vi "ScanTrans.vi"(0 "Type of scan":u16(ring)=3 items=["Therapy With Scan", "M scan", "M Scan With Therapy Burst", "1-D B Scan", "1-D B Scan With Therapy Burst", "2-D B Scan", "2-D B Scan With Therapy Burst", "Rotational Scan", "1-D B-Scan PRF", "2-D B-Scan PRF", "Real-Time Scan", "Contrast Agents", "1-D w/ Real-Time Set Up", "Amplifier blah blah"], 1 "File Name":string, 2 "Digitizer Settings":T5={"Digitizer delay (us) "=0.0, "rf points per line"=2048, "lines per plane"=128, "Samp Rate (Hz)"=100000000.0, "Additional dig delay (us)"=0.0, "Voltage Scale"=0.4, "Pre-Looks"=0, "Offset delay (us)"=0.0, "bits A/D"=8, "Avg Num"=1, "DigTimeOut"=5.0, "Rel Dig Delay"=0.0, "Dig Ch"=0, "LeCroyCluster"={"LeCroy Channels"=[TRUE, FALSE, FALSE, FALSE], "LC read pt offset"=0.0, "Sweep Avg"=FALSE}, "Main Digitizer"=enum."NI Digitizer", "Dig Config"=enum."Single channel", "Digitizer ID Cluster"={"Acqiris/Alazar/SP ID"=[], "NI Instr Handles"=[], "LeCroy VISA"="", "GaGe Handle"={"Handle"=0, "Sample size"=0, "Resolution"=0, "Offset"=0, "Channels"=0, "Boards"=0}, "ATS Ref"="ATS9350", "Acqiris Address"=["PCI::INSTR0"], "ADQRef"=refnum, "adq_cu_ptr"=refnum}, "Trigger Settings"={"Trig Source"=1, "Trig Coupling"=0, "Trig Slope"=0, "Level (mV)"=1500.0}, "Bulk Acq"=FALSE, "Bulk Start Indexes"=[], "Data Ref RF"=refnum, "NI ID/Channel"=[], "Total Dig CH"=5, "Xtra Ann Trig delay (us)"=10.0, "Fix Z Delay?"=FALSE, "One Way Transmission?"=FALSE, "Data Ref Log"=refnum} {"Trigger Settings"."Trig Slope" items=["Positive", "Negative"]; "Trigger Settings"."Level (mV)" format="%.2f"; "Trigger Settings"."Trig Coupling" items=["DC 1 MOhm", "AC 1 MOhm", "DC 50 Ohm", "AC 50 Ohm"]; "Trigger Settings"."Trig Source" items=["Chan 1", "External"]; "Rel Dig Delay" format="%.2f"; "DigTimeOut" format="%.2f"; "Avg Num" min=1; "Offset delay (us)" format="%.2f"; "Additional dig delay (us)" format="%.2f"; "Digitizer delay (us)" format="%.2f"}, 5 "Scan Length (mm)":dbl=10.0 format="%.2f", 7 "Therapy":bool, 12 "Motion Settings":T1={"No Motion?"=FALSE, "Motion System"=enum."No Motion Card", "Motion Bd ID"=1, "Motion Profile"="SMAC1", "# Axis"=1, "Reverse Z axis?"=TRUE, "SMAC Axis"=0, "scan pair"=enum."y-(x) scan", "RT fps"=6.0, "Steps per mm"=[1000, 1000, 1000, 1000], "Motor Parameters"={"velocity ct/s"=[10000.0, 10000.0, 10000.0, 50000.0], "accel ct/s^2"=[50000.0, 50000.0, 50000.0, 200000.0]}, "One Way Scan"=FALSE, "Reverse One Way Scan"=FALSE, "Global Position (mm)"=[], "Plane"=0, "Distance between\nscan lines (um)"=0.0, "Distance between\nscan planes (um)"=0.0, "number of scan planes"=1, "Total steps in line"=0, "Xtra plane\ndistance  (um)"=100, "Xtra planes "=1, "Add Axis"=FALSE, "overshoot cts"=200, "BKPT Shift"=0, "Scan Start Time (ms)"=0, "ESP VISA"="GPIB::1::INSTR", "3rd Axis"=1, "GL Ref Out"=refnum, "Galil Address"=""} {"3rd Axis" items=["x", "y", "z", "w"]; "Xtra planes" min=1; "Xtra plane\ndistance  (um)" min=0; "Distance between\nscan planes (um)" format="%.2f"; "Distance between\nscan lines (um)" format="%.2f"; "SMAC Axis" items=["None"=0, "Axis 1"=1, "Axis 2"=2, "Axis 3"=3, "Axis 4"=4, "Axis 5"=5, "Axis 6"=6, "Axis 7"=7, "Axis 8"=8, "Vector Space 1"=17, "Vector Space 2"=18, "Vector Space 3"=19, "Vector Space 4"=20]; "Motion Bd ID" min=1 max=32 step=1}, 14 "Pressure Cal Parameters":T9={"Center Freq (MHz)"=0.0, "PRF (kHz)"=0.0, "Pulse window (us)"=0.0, "Hydrophone"=enum."PAL #1048", "booster amp?"=TRUE} {"Pulse window (us)" format="%.2f"; "PRF (kHz)" format="%.2f"; "Center Freq (MHz)" format="%.2f"}) -> (4 "Scan data":T11 {"Pulse Parameters"."pos peak pressure (MPa)" format="%.2f"; "axis 2 ticks" format="%.2f"; "axis 1 ticks" format="%.2f"; "step size" format="%.2f"; "axis2o" format="%.2f"; "axis1o" format="%.2f"; "scan data" format="%.2f"})   [LabVIEW 2022 SP3]
uses:
  HydrophoneSettings.ctl
  Hydros.ctl
  ScanningControl/Digitizers/-DigitizerRoutines/DigitizerSettings.ctl
  ScanningControl/Digitizers/-DigitizerRoutines/Digitizer.ctl
  ScanningControl/Digitizers/-DigitizerRoutines/DigConfig.ctl
  ScanningControl/Digitizers/-DigitizerRoutines/DigitizerID.ctl
  C:/Windows/System32/ADQAPI_dotNet_helper.dll
  ScanningControl/Motion Controllers/NI_controller/-NI_MotionRoutines/MotionParameters.ctl
  ScanningControl/Motion Controllers/NI_controller/-NI_MotionRoutines/MotionSys.ctl
  ScanningControl/Motion Controllers/-MotionRoutines/ScanAxis.ctl
  ScanningControl/Motion Controllers/-MotionRoutines/3rdAxis.ctl
  ScanningControl/Motion Controllers/-MotionRoutines/MotionGlobals.vi
panel:
  out "Waveform Graph":dbl[](graph)
  # "1-D and 2-D B scan settings"
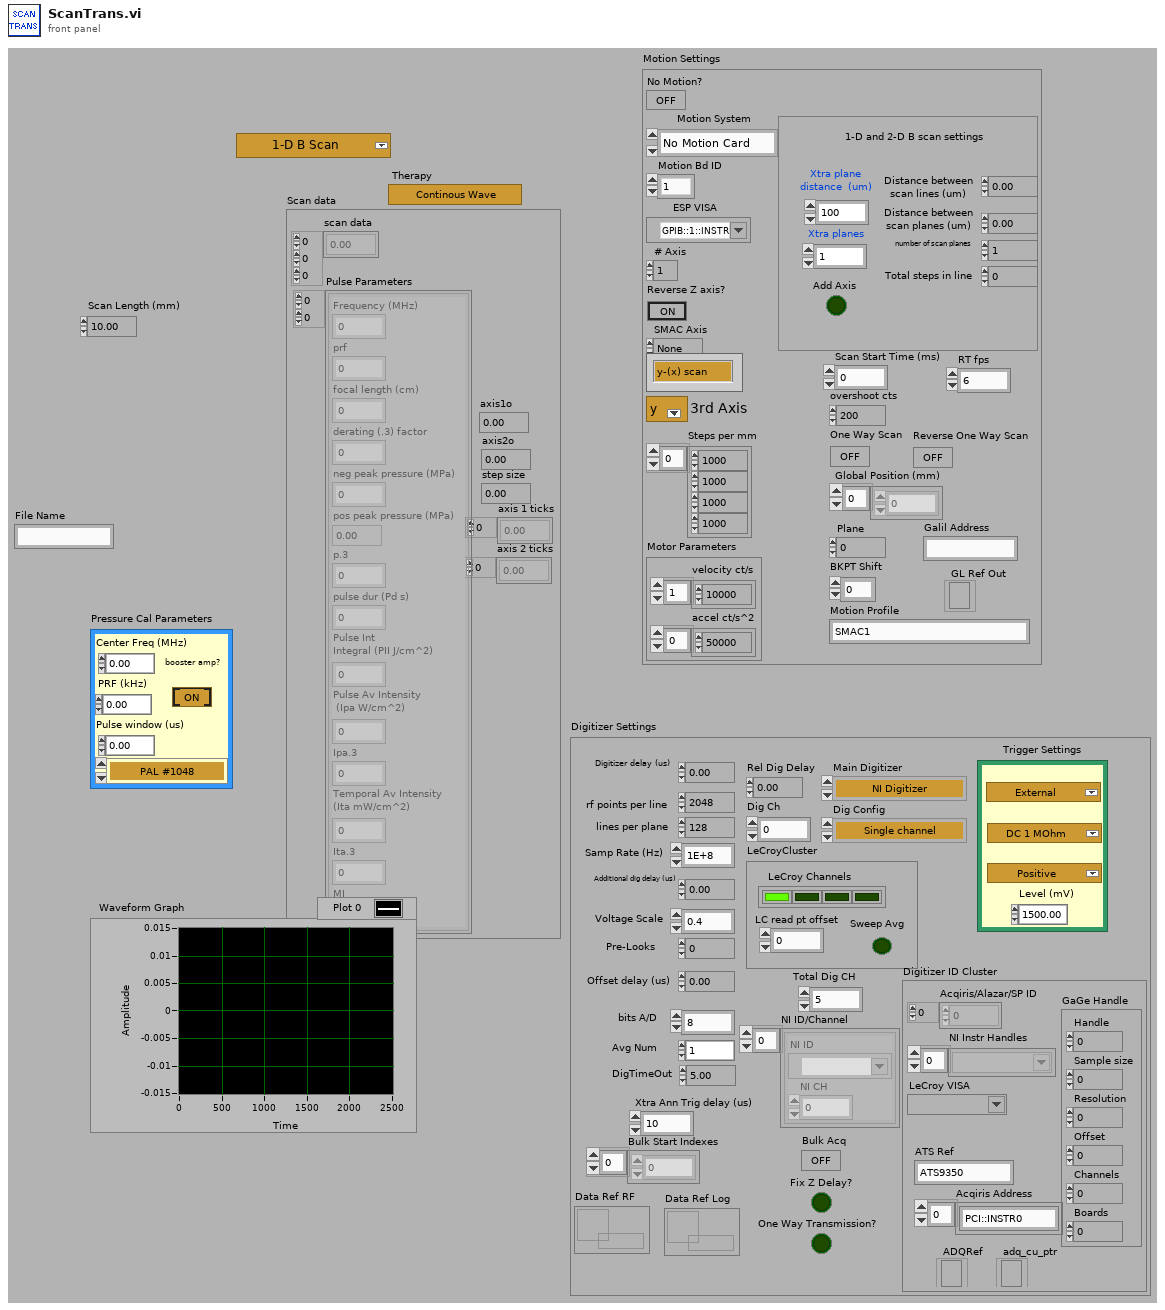
[diagram p1: front panel]
types:
  T1 = typedef "MotionParameters.ctl" = cluster{"No Motion?":bool, "Motion System":T2, "Motion Bd ID":u8, "Motion Profile":string, "# Axis":i8, "Reverse Z axis?":bool, "SMAC Axis":u16, "scan pair":T3, "RT fps":sgl, "Steps per mm":i32[], "Motor Parameters":cluster{"velocity ct/s":dbl[], "accel ct/s^2":dbl[]}, "One Way Scan":bool, "Reverse One Way Scan":bool, "Global Position (mm)":dbl[], "Plane":i32, "Distance between\nscan lines (um)":sgl, "Distance between\nscan planes (um)":sgl, "number of scan planes":i32, "Total steps in line":i32, "Xtra plane\ndistance  (um)":i32, "Xtra planes ":i32, "Add Axis":bool, "overshoot cts":i32, "BKPT Shift":i32, "Scan Start Time (ms)":u32, "ESP VISA":refnum<visa-resource-name>, "3rd Axis":T4, "GL Ref Out":refnum<k7>, "Galil Address":string}
  T2 = typedef "MotionSys.ctl" = enum16{"MM3000", "NI 735x", "Newport ESP", "No Motion Card", "Galil"}
  T3 = typedef "ScanAxis.ctl" = enum16{"y-(x) scan", "x-(y) scan", "z-(x) scan", "z-(y) scan", "y-(z) scan", "x-(z) scan", "w-(x) scan", "w-(y) scan", "w-(z) scan", "x-(w) scan", "y-(w) scan", "z-(w) scan"}
  T4 = typedef "3rdAxis.ctl" = u16
  T5 = typedef "DigitizerSettings.ctl" = cluster{"Digitizer delay (us) ":dbl, "rf points per line":i32, "lines per plane":i32, "Samp Rate (Hz)":dbl, "Additional dig delay (us)":dbl, "Voltage Scale":dbl, "Pre-Looks":i32, "Offset delay (us)":dbl, "bits A/D":i8, "Avg Num":i32, "DigTimeOut":sgl, "Rel Dig Delay":sgl, "Dig Ch":i32, "LeCroyCluster":cluster{"LeCroy Channels":bool[], "LC read pt offset":dbl, "Sweep Avg":bool}, "Main Digitizer":T6, "Dig Config":T7, "Digitizer ID Cluster":T8, "Trigger Settings":cluster{"Trig Source":u16, "Trig Coupling":u16, "Trig Slope":u16, "Level (mV)":dbl}, "Bulk Acq":bool, "Bulk Start Indexes":i32[], "Data Ref RF":refnum<data-value>, "NI ID/Channel":cluster{"NI ID":refnum<k15>, "NI CH":i32}[], "Total Dig CH":i32, "Xtra Ann Trig delay (us)":dbl, "Fix Z Delay?":bool, "One Way Transmission?":bool, "Data Ref Log":refnum<data-value>}
  T6 = typedef "Digitizer.ctl" = enum16{"Acqiris Digitizer", "NI Digitizer", "LeCroy", "GaGe", "AlazarTech", "No Digitizer", "Teledyne"}
  T7 = typedef "DigConfig.ctl" = enum16{"Single channel", "2 Chans w/ 2 Acqiris", "2 Chans w/ 1 Acqiris", "5-CH Pulser New", "5-CH pulser w/ ann array", "5-pass style ann array", "Empty"}
  T8 = typedef "DigitizerID.ctl" = cluster{"Acqiris/Alazar/SP ID":u32[], "NI Instr Handles":refnum<k15>[], "LeCroy VISA":refnum<visa-resource-name>, "GaGe Handle":cluster{"Handle":u32, "Sample size":u32, "Resolution":i32, "Offset":i32, "Channels":u32, "Boards":u32}, "ATS Ref":string, "Acqiris Address":string[], "ADQRef":refnum<k24>, "adq_cu_ptr":refnum<k24>}
  T9 = typedef "HydrophoneSettings.ctl" = cluster{"Center Freq (MHz)":dbl, "PRF (kHz)":dbl, "Pulse window (us)":dbl, "Hydrophone":T10, "booster amp?":bool}
  T10 = typedef "Hydros.ctl" = enum16{"PAL #1048", "PAL #525", "PAL #430a", "PAL #192", "DEAD PAL # 1403", "LOST UHI Onda", "DEAD PAL #1818", "PAL #1974", "DEAD #2266 w/booster", "PAL #2524 w/booster", "PAL FP21-20T", "PAL FP160-13  ", "PAL FP141-20", "PAL FP158-08T"}
  T11 = cluster{"scan data":dbl[][][], "Pulse Parameters":cluster{"Frequency (MHz)":dbl, "prf":dbl, "focal length (cm)":dbl, "derating (.3) factor":dbl, "neg peak pressure (MPa)":dbl, "pos peak pressure (MPa)":dbl, "p.3":dbl, "pulse dur (Pd s)":dbl, "Pulse Int \nIntegral (PII J/cm^2)":dbl, "Pulse Av Intensity\n (Ipa W/cm^2)":dbl, "Ipa.3":dbl, "Temporal Av Intensity \n(Ita mW/cm^2)":dbl, "Ita.3":dbl, "MI":dbl}[][], "axis1o":dbl, "axis2o":dbl, "step size":dbl, "axis 1 ticks":dbl[], "axis 2 ticks":dbl[]}
  T12 = enum16{"Absolute Position", "Relative Position", "Velocity", "Relative to Cap Pos", "Modulus Position", "Absolute Contouring", "Relative Contouring"}
  T13 = cluster{"Frequency (MHz)":dbl, "prf":dbl, "focal length (cm)":dbl, "derating (.3) factor":dbl, "neg peak pressure (MPa)":dbl, "pos peak pressure (MPa)":dbl, "p.3":dbl, "pulse dur (Pd s)":dbl, "Pulse Int \nIntegral (PII J/cm^2)":dbl, "Pulse Av Intensity\n (Ipa W/cm^2)":dbl, "Ipa.3":dbl, "Temporal Av Intensity \n(Ita mW/cm^2)":dbl, "Ita.3":dbl, "MI":dbl}[][]
  T14 = cluster{"Axis 1 Start":dbl, "Axis 2 Start":dbl, "Step Size":dbl, "Axis 1 Ticks":dbl[], "Axis 2 Ticks":dbl[]}
  T15 = cluster{dbl[][][], "Data":cluster{"Frequency (MHz)":dbl, "prf":dbl, "focal length (cm)":dbl, "derating (.3) factor":dbl, "neg peak pressure (MPa)":dbl, "pos peak pressure (MPa)":dbl, "p.3":dbl, "pulse dur (Pd s)":dbl, "Pulse Int \nIntegral (PII J/cm^2)":dbl, "Pulse Av Intensity\n (Ipa W/cm^2)":dbl, "Ipa.3":dbl, "Temporal Av Intensity \n(Ita mW/cm^2)":dbl, "Ita.3":dbl, "MI":dbl}[][], "Axis 1 Start":dbl, "Axis 2 Start":dbl, "Step Size":dbl, "Axis 1 Ticks":dbl[], "Axis 2 Ticks":dbl[]}
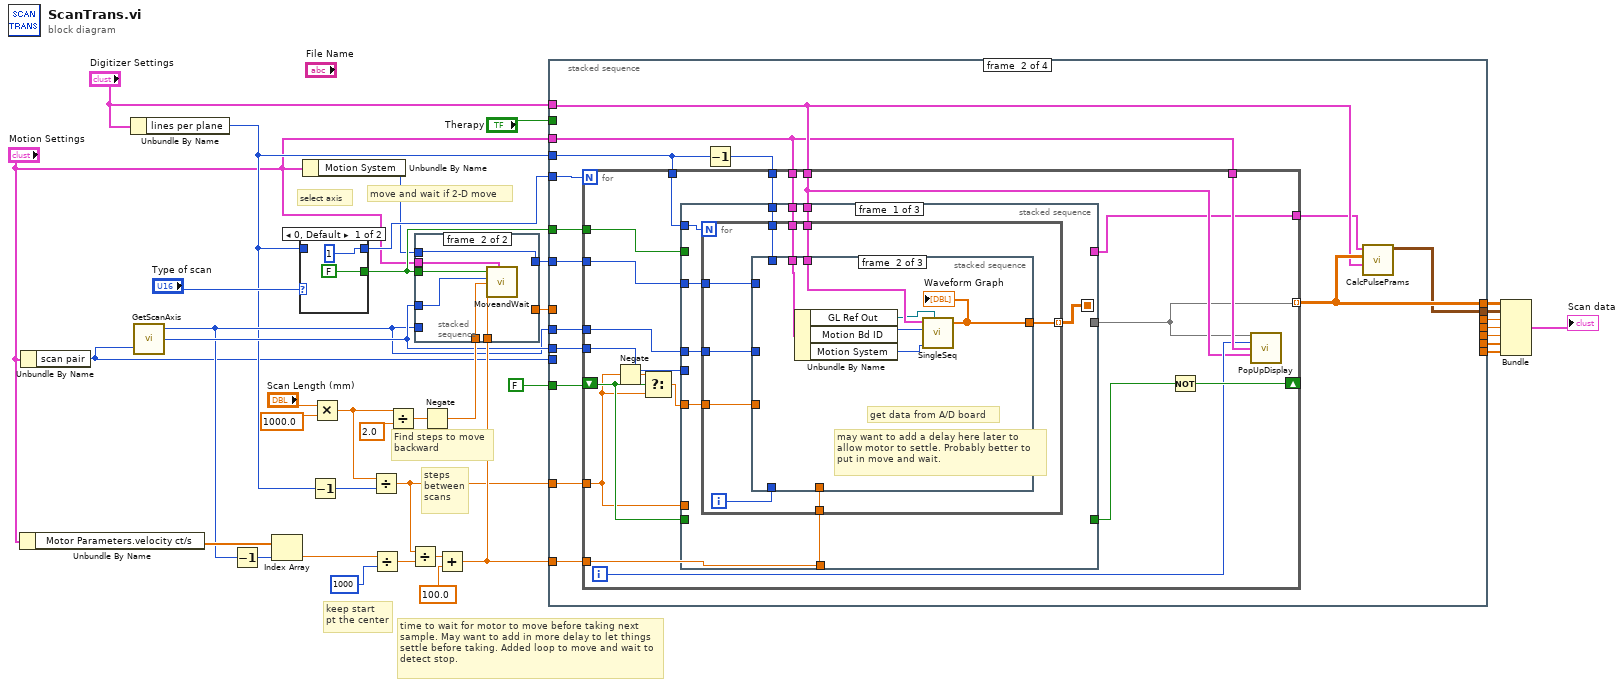
[diagram p0: block diagram]
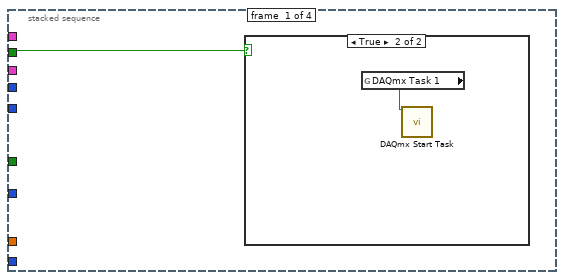
[diagram p2: hidden frame]
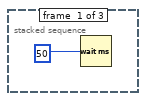
[diagram p4: hidden frame]
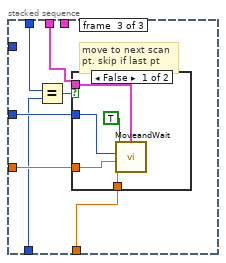
[diagram p5: hidden frame]
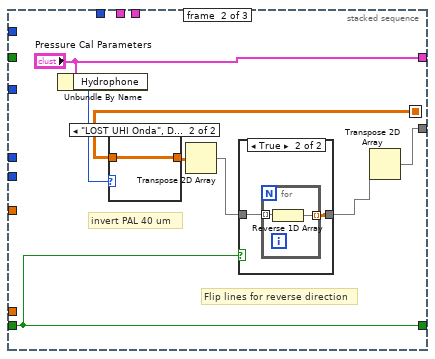
[diagram p7: hidden frame]
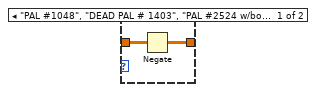
[diagram p9: hidden frame]
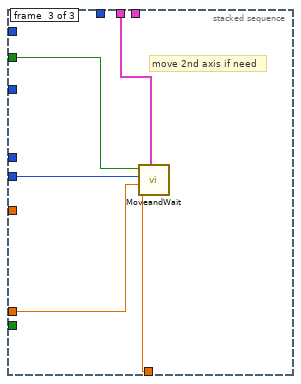
[diagram p10: hidden frame]
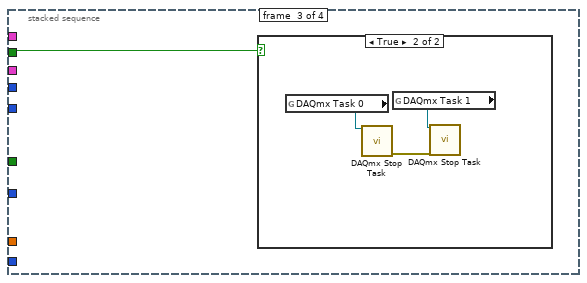
[diagram p11: hidden frame]
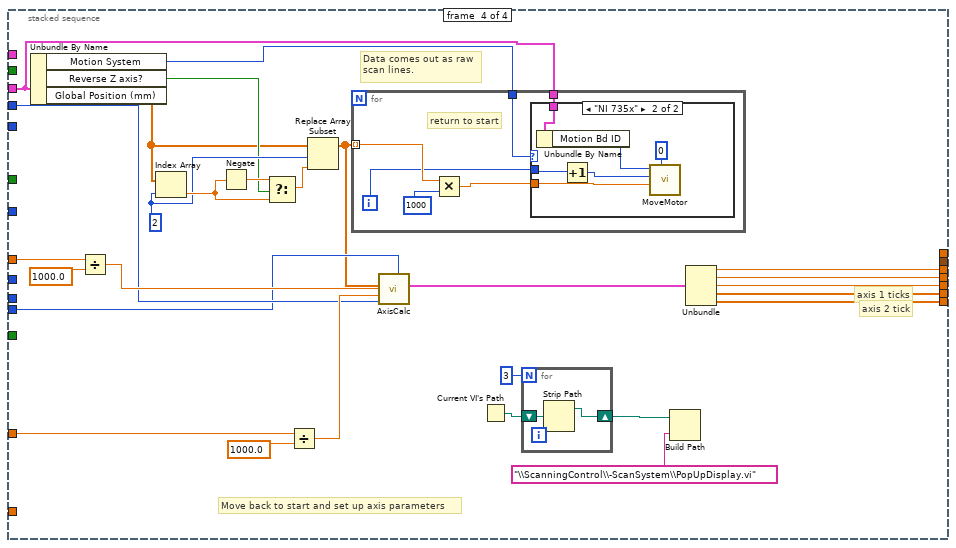
[diagram p13: hidden frame]
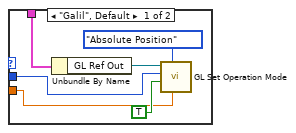
[diagram p14: hidden frame]
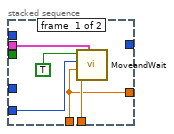
[diagram p15: hidden frame]
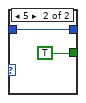
[diagram p16: hidden frame]
diagram:
  # "steps\nbetween\nscans"
  # "Find steps to move\nbackward"
  # "select axis"
  # "move and wait if 2-D move"
  # "time to wait for motor to move before taking next sample. May want to add in more delay to let things settle before taking. Added loop to move and wait to detect stop."
  # "keep start\npt the center"
  n1 = Unbundle By Name("Motion Settings") -> ("Motor Parameters.velocity ct/s"=w9:dbl[])
  n2 = Unbundle By Name("Motion Settings") -> ("scan pair"=w4:T3)
  n3 = Unbundle By Name("Digitizer Settings") -> ("lines per plane"=w5:i32)
  n4 = call "GetScanAxis.vi"("scan pair"=w4) -> ("Axis 1"=w7:i32, "Axis 2"=w11:i32)  [unwired: 1 in, 1 out]
  n5 = Decrement(x=w7) -> (x-1=w6:i32)
  n6 = Index Array(array=w9, index=w6) -> (element=w8:dbl)
  n7 = case shown="0, Default" "Type of scan" {
    tunnel: [1 w41] -> w37
    tunnel: w5 -> [_ w41]
    tunnel: [FALSE TRUE] -> w25
    frame 0, Default {
    }
    frame 5 {
      # "y"
    }
  }
  n8 = Unbundle By Name("Motion Settings") -> ("Motion System"=w3:T2)
  n9 = Decrement(x=w5) -> (x-1=w29:i32)
  n10 = Multiply(x="Scan Length (mm)", y=1000.0) -> (x*y=w30:dbl)
  n11 = Divide(x=w30, y=w29) -> (x/y=w22:dbl)
  n12 = Divide(x=w8, y=1000) -> (x/y=w27:dbl)
  n13 = Divide(x=w30, y=2.0) -> (x/y=w32:dbl)
  n14 = Divide(x=w22, y=w27) -> (x/y=w35:dbl)
  n15 = Negate(x=w32) -> (-x=w23:dbl)
  n16 = Add(x=w35, y=100.0) -> (x+y=w26:dbl)
  n17 = stacked-sequence {
    tunnel: w25 -> [_ w53]
    tunnel: w11 -> [_ w52]
    tunnel: w23 -> [w45 w51]
    tunnel: w26 -> [w46 w50]
    tunnel: w7 -> [w44 _]
    tunnel: [w45 _] -> w20
    tunnel: w3 -> [_ w49]
    tunnel: [_ w49] -> w19
    tunnel: "Motion Settings" -> [w43 w48]
    frame #0 {
      n18 = call "MoveandWait.vi"("Motion Settings"=w43, "time to wait (ms)"=w46, "steps to move"=w45, "Axis"=w44, "Move and Wait?"=TRUE) -> ()  [unwired: 1 in, 2 out]
    }
    frame #1 {
      n19 = call "MoveandWait.vi"("Motion Settings"=w48, "time to wait (ms)"=w50, "steps to move"=w51, "Axis"=w52, "Move and Wait?"=w53) -> ()  [unwired: 1 in, 2 out]
    }
  }
  n20 = stacked-sequence {
    tunnel: w37 -> [_ w70 _ _]
    tunnel: FALSE -> [_ w69 _ _]
    tunnel: w26 -> [_ w67 _ _]
    tunnel: w7 -> [_ w66 _ _]
    tunnel: w25 -> [_ w65 _ _]
    tunnel: w11 -> [_ w64 _ _]
    tunnel: w22 -> [_ w63 _ w176]
    tunnel: [_ w60 _ _] -> w24
    tunnel: w5 -> [_ w62 _ w165]
    tunnel: [_ w59 _ _] -> w21
    tunnel: w20 -> [_ _ _ w174]
    tunnel: w19 -> [_ w61 _ _]
    tunnel: [_ _ _ w172] -> w18
    tunnel: [_ _ _ w171] -> w17
    tunnel: [_ _ _ w170] -> w16
    tunnel: [_ _ _ w169] -> w15
    tunnel: [_ _ _ w168] -> w14
    tunnel: "Therapy" -> [w54 _ w148 _]
    tunnel: w4 -> [_ _ _ w164]
    tunnel: "Digitizer Settings" -> [_ w58 _ _]
    tunnel: "Motion Settings" -> [_ w56 _ w152]
    frame #0 {
      n21 = case shown="True" w54 {
        frame False {
        }
        frame True {
          n22 = global read "MotionGlobals.vi" "DAQmx Task 1"() -> (w55:refnum<k21>)
          n23 = call <vilib>:"DAQmx Start Task.vi"("task/channels in"=w55) -> ()  [unwired: 1 in, 14 out]
        }
      }
    }
    frame #1 {
      n24 = Decrement(x=w62) -> (x-1=w68:i32)
      n25 = for {
        N: w70 -> [_]
        tunnel: w66 -> [w85]
        tunnel: w62 -> [w89]
        shift-right: [w88] -> _
        shift-left: w69 -> [w81]
        tunnel: w63 -> [w79]
        tunnel: w67 -> [w82]
        tunnel: w68 -> [w86]
        tunnel: w65 -> [w84]
        tunnel: w64 -> [w83]
        tunnel: [w72] -> w60 mode=indexing
        tunnel: w61 -> [w77]
        tunnel: w58 -> [w74]
        tunnel: w56 -> [w76]
        tunnel: [w73] -> w57
        tunnel: w56 -> [w71]
        i -> [w75]
        n26 = Negate(x=w79) -> (-x=w78:dbl)
        n27 = Select(t=w78, s=w81, f=w79) -> (s? t:f=w87:dbl)
        n28 = stacked-sequence {
          seq-local: [w91 _ _] -> [_ w132 _]
          tunnel: w89 -> [w98 _ _]
          tunnel: w87 -> [w94 _ _]
          tunnel: w86 -> [w97 _ _]
          tunnel: [_ w127 _] -> w72
          tunnel: w82 -> [w96 _ w145]
          tunnel: w85 -> [w95 _ _]
          tunnel: w84 -> [_ _ w147]
          tunnel: w83 -> [_ _ w146]
          tunnel: w79 -> [_ _ w144]
          tunnel: w81 -> [_ w129 _]
          tunnel: [_ w129 _] -> w80
          tunnel: w77 -> [w93 _ _]
          tunnel: w74 -> [w92 _ _]
          tunnel: [_ "Pressure Cal Parameters" _] -> w73
          tunnel: w71 -> [w90 _ w143]
          frame #0 {
            n29 = for {
              N: w98 -> [_]
              tunnel: w95 -> [w107]
              tunnel: w94 -> [w106]
              tunnel: w96 -> [w105]
              tunnel: w97 -> [w104]
              tunnel: [w102] -> w91 mode=indexing
              tunnel: w93 -> [w101]
              tunnel: w92 -> [w100]
              tunnel: w90 -> [w99]
              i -> [w103]
              n30 = stacked-sequence {
                tunnel: w107 -> [_ _ w121]
                tunnel: w106 -> [_ _ w120]
                tunnel: w105 -> [_ _ w116]
                tunnel: w104 -> [_ _ w119]
                tunnel: w103 -> [_ _ w118]
                tunnel: [_ w114 _] -> w102
                tunnel: w101 -> [_ _ _]
                tunnel: w100 -> [_ w113 _]
                tunnel: w99 -> [_ w112 w115]
                frame #0 {
                  n31 = Wait (ms)(milliseconds to wait=50) -> ()  [unwired: 1 out]
                }
                frame #1 {
                  # "may want to add a delay here later to\nallow motor to settle. Probably better to\nput in move and wait."
                  # "get data from A/D board"
                  n32 = Unbundle By Name(w112) -> ("GL Ref Out"=w109:refnum<k7>, "Motion Bd ID"=w110:u8, "Motion System"=w111:T2)
                  n33 = call "SingleSeq.vi"("Motion System"=w111, "GL Ref Out"=w109, "Motion Bd ID"=w110, "Digitizer Settings"=w113) -> ("waveform"=w114:dbl[])  [unwired: 2 in, 4 out]
                  "Waveform Graph" <- w114
                }
                frame #2 {
                  # "move to next scan\npt. skip if last pt"
                  n34 = Equal?(x=w119, y=w118) -> (x = y?=w117:bool)
                  n35 = case shown="False" w117 {
                    tunnel: w121 -> [w124 _]
                    tunnel: w120 -> [w126 _]
                    tunnel: w116 -> [w125 _]
                    tunnel: w115 -> [w122 _]
                    frame False {
                      n36 = call "MoveandWait.vi"("Motion Settings"=w122, "time to wait (ms)"=w125, "steps to move"=w126, "Axis"=w124, "Move and Wait?"=TRUE) -> ()  [unwired: 1 in, 2 out]
                    }
                    frame True {
                    }
                  }
                }
              }
            }
          }
          frame #1 {
            # "invert PAL 40 um"
            # "Flip lines for reverse direction"
            n37 = Unbundle By Name("Pressure Cal Parameters") -> ("Hydrophone"=w134:T10)
            n38 = case shown="\"LOST UHI Onda\", Default" w134 {
              tunnel: w132 -> [w141 w142]
              tunnel: [w140 w142] -> w131
              frame "PAL #1048", "DEAD PAL # 1403", "PAL #2524 w/booster" {
                n39 = Negate(x=w141) -> (-x=w140:dbl[][])
              }
              frame "LOST UHI Onda", Default {
              }
            }
            n40 = Transpose 2D Array(2D array=w131) -> (transposed array=w130:dbl[][])
            n41 = case shown="True" w129 {
              tunnel: [w135 w137] -> w128
              tunnel: w130 -> [w135 w136]
              frame False {
              }
              frame True {
                n42 = for {
                  tunnel: w136 -> [w139] mode=indexing
                  tunnel: [w138] -> w137 mode=indexing
                  n43 = Reverse 1D Array(array=w139) -> (reversed array=w138:dbl[])
                }
              }
            }
            n44 = Transpose 2D Array(2D array=w128) -> (transposed array=w127:dbl[][])
          }
          frame #2 {
            # "move 2nd axis if need"
            n45 = call "MoveandWait.vi"("Motion Settings"=w143, "time to wait (ms)"=w145, "steps to move"=w144, "Axis"=w146, "Move and Wait?"=w147) -> ()  [unwired: 1 in, 2 out]
          }
        }
        n46 = Not(x=w80) -> (.not. x?=w88:bool)
        n47 = call "PopUpDisplay.vi"("Data"=w72, "Plane"=w75, "Motion Settings In"=w76, "Digitizer Settings"=w74) -> ()  [unwired: 12 in]
      }
      n48 = call "CalcPulsePrams.vi"("Digitizer Settings"=w58, "Array"=w60, "Pressure Cal Parameters"=w57) -> ("Data"=w59:T13)  [unwired: 8 in]
    }
    frame #2 {
      n49 = case shown="True" w148 {
        frame False {
        }
        frame True {
          n50 = global read "MotionGlobals.vi" "DAQmx Task 0"() -> (w149:refnum<k21>)
          n51 = call <vilib>:"DAQmx Stop Task.vi"("task/channels in"=w149) -> ("error out"=w151:errorcluster)  [unwired: 1 in, 13 out]
          n52 = global read "MotionGlobals.vi" "DAQmx Task 1"() -> (w150:refnum<k21>)
          n53 = call <vilib>:"DAQmx Stop Task.vi"("task/channels in"=w150, "error in"=w151) -> ()  [unwired: 14 out]
        }
      }
    }
    frame #3 {
      w161 = 2 ("index")
      # "Data comes out as raw\nscan lines."
      # "Move back to start and set up axis parameters"
      # "axis 1 ticks"
      # "axis 2 tick"
      n54 = Unbundle By Name(w152) -> ("Motion System"=w153:T2, "Reverse Z axis?"=w160:bool, "Global Position (mm)"=w159:dbl[])
      n55 = Divide(x=w174, y=1000.0) -> (x/y=w166:dbl)
      n56 = Index Array(array=w159, index=w161) -> (element=w163:dbl)
      n57 = Negate(x=w163) -> (-x=w175:dbl)
      n58 = Select(t=w175, s=w160, f=w163) -> (s? t:f=w162:dbl)
      n59 = Divide(x=w176, y=1000.0) -> (x/y=w167:dbl)
      n60 = Replace Array Subset(array=w159, new element=w162, index=w161) -> (w158:dbl[])
      n61 = for {
        tunnel: w158 -> [w184] mode=indexing
        tunnel: w153 -> [w183]
        tunnel: w152 -> [w182]
        i -> [w181]
        # "return to start"
        n62 = Multiply(x=w184, y=1000) -> (x*y=w186:dbl)
        n63 = case shown="\"NI 735x\"" w183 {
          tunnel: w186 -> [w188 w198]
          tunnel: w182 -> [w189 w196]
          tunnel: w181 -> [w187 w194]
          frame "Galil", Default {
            n64 = Unbundle By Name(w189) -> ("GL Ref Out"=w191:refnum<k7>)
            n65 = call "GL Set Operation Mode.vi"("position cts (abs/rel)"=w188, "Position Mode (Absolute)"=T12."Absolute Position", "Start Now?"=TRUE, "Axis"=w187, "Galil.IGalil"=w191) -> ()  [unwired: 4 in, 3 out]
          }
          frame "NI 735x" {
            n66 = Unbundle By Name(w196) -> ("Motion Bd ID"=w195:u8)
            n67 = Increment(x=w194) -> (x+1=w193:i32)
            n68 = call "MoveMotor.vi"("Position Mode (Absolute)"=0, "Target Position (0)"=w198, "Axis or Vector Space"=w193, "Motion Bd ID"=w195) -> ()  [unwired: 1 in, 7 out]
          }
        }
      }
      n69 = call "AxisCalc.vi"("ScanAxis"=w164, "start"=w166, "Number of pts\nper scan"=w165, "increment"=w167, "Global Position (mm)"=w158) -> ("axis"=w173:T14)  [unwired: 2 in, 4 out]
      n70 = Current VI's Path() -> (path=w157:path)
      n71 = for {
        N: 3 -> [_]
        shift-right: [w179] -> w155
        shift-left: w157 -> [w180]
        n72 = Strip Path(path=w180) -> (stripped path=w179:path)  [unwired: 1 out]
      }
      n73 = Build Path(base path=w155, name or relative path="\\ScanningControl\\-ScanSystem\\PopUpDisplay.vi") -> ()  [unwired: 1 out]
      n74 = Unbundle(w173) -> ("Axis 1 Start"=w172:dbl, "Axis 2 Start"=w171:dbl, "Step Size"=w170:dbl, "Axis 1 Ticks"=w169:dbl[], "Axis 2 Ticks"=w168:dbl[])
    }
  }
  n75 = Bundle(w24, "Data"=w21, "Axis 1 Start"=w18, "Axis 2 Start"=w17, "Step Size"=w16, "Axis 1 Ticks"=w15, "Axis 2 Ticks"=w14) -> (→"Scan data":T15)  [unwired: 1 out]
